vi "LS330_Set_Setpoint&Ramp_DP_ver1.0.vi"(5 "Mode: (default: 2)":i16(ring)=2 items=["Do nothing to mark the end of the transfer", "Send NL (linefeed) with EOI after the data bytes.", "Send EOI with the last data byte in the string(default)"], 6 "Ramping Enable (T)":bool=TRUE, 8 "error in":errorcluster, 9 "Ramping rate (0-100 K/min; 1.0)":dbl=1.0 format="%.3f", 10 "Setpoint (2-400 K)":dbl=2.0 min=2.0 max=400.0 format="%.3f", 11 "GPIB ADR (19)":i16=19) -> (0 "error out":errorcluster, 3 "dump GPIB ADR":i16)   [LabVIEW 2012]
doc: "This VI configures the Setpoint and Setpoint Ramping function. The Setpoint parameter is used to set the desired load temperature for a control loop.\nTotal delay would be 1 sec"
uses:
  Instance           2 38Saved   LS330_Set_Setpoint&Ramp_ver1.0 .vi
  Instance           1 38Saved   LS330_Set_Setpoint&Ramp_ver1.0 .vi
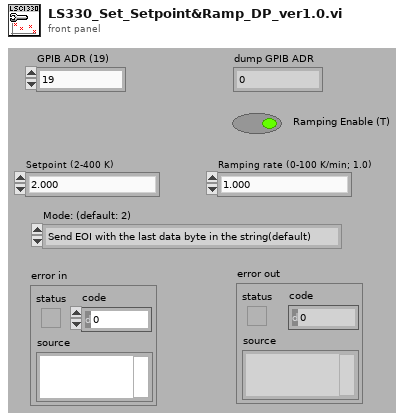
[diagram p1: front panel]
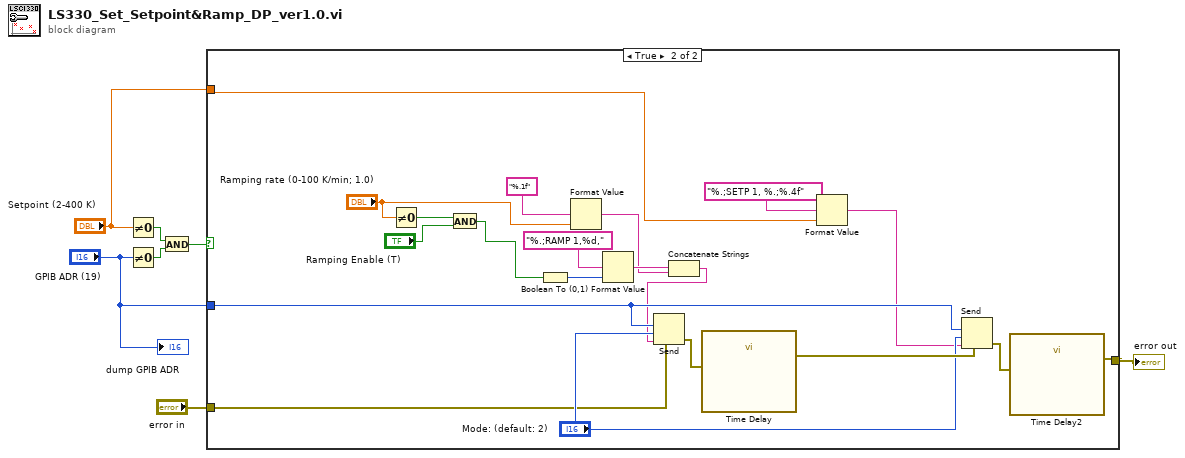
[diagram p0: block diagram]
diagram:
  n1 = Not Equal To 0?(x="Setpoint (2-400 K)") -> (x != 0?=w3:bool)
  n2 = Not Equal To 0?(x="GPIB ADR (19)") -> (x != 0?=w4:bool)
  n3 = And(x=w3, y=w4) -> (x .and. y?=w2:bool)
  n4 = case shown="True" w2 {
    tunnel: "GPIB ADR (19)" -> [_ w25]
    tunnel: "error in" -> [w8 w24]
    tunnel: [w8 w23] -> w6
    tunnel: "Setpoint (2-400 K)" -> [_ w22]
    frame False {
    }
    frame True {
      n5 = Not Equal To 0?(x="Ramping rate (0-100 K/min; 1.0)") -> (x != 0?=w17:bool)
      n6 = And(x=w17, y="Ramping Enable (T)") -> (x .and. y?=w18:bool)
      n7 = Boolean To (0,1)(Boolean=w18) -> (0, 1=w13:i16)
      n8 = Format Value(format string="%.1f", value (0)="Ramping rate (0-100 K/min; 1.0)") -> (output string=w10:string)  [unwired: 1 in]
      n9 = Format Value(format string="%.;RAMP 1,%d,", value (0)=w13) -> (output string=w11:string)  [unwired: 1 in]
      n10 = Concatenate Strings(w11, w10) -> (w9:string)
      n11 = Send(2:w25, 3:"Mode: (default: 2)", 4:w24, 5:w9) -> (8:w19:errorcluster)  [unwired: 1 in, 2 out]
      n12 = call "Time Delay"("error in (no error)"=w19) -> ("error out"=w28:errorcluster)  [unwired: 10 in]
      n13 = Format Value(format string="%.;SETP 1, %.;%.4f", value (0)=w22) -> (output string=w21:string)  [unwired: 1 in]
      n14 = Send(2:w25, 3:"Mode: (default: 2)", 4:w28, 5:w21) -> (8:w27:errorcluster)  [unwired: 1 in, 2 out]
      n15 = call "Time Delay2"("error in (no error)"=w27) -> ("error out"=w23:errorcluster)  [unwired: 10 in]
    }
  }
  "error out" <- w6
  "dump GPIB ADR" <- "GPIB ADR (19)"
